vi "Attitude Control Test.vi"() -> ()   [LabVIEW 2022 SP3]
doc: "This example is used to make the attitude control"
uses:
  <vilib>/Utility/miscctls.llb/LV3DPointTypeDef.ctl
  lv-attitudecontrol.lvlib
panel:
  out "Numeric 3":dbl
  out "Numeric 2":dbl
  out "Numeric":dbl
  in  "Attitude Indicator":refnum<vi>(3d-picture)
  in  "stop":bool
  in  "Control 1":T1 {"X" scale=-90.0..90.0; "Y" scale=-180.0..180.0; "Z" scale=0.0..360.0}
  # "Overview: This example is used to make the attitude control\nRequirements: LabVIEW 2012 (or compatible)\nInstructions: \n1. Run this VI"
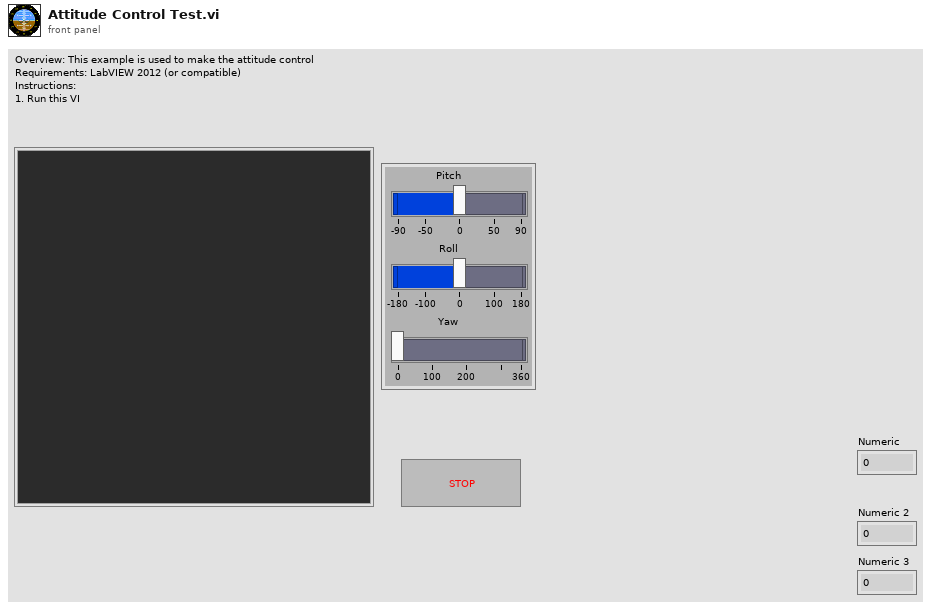
[diagram p1: front panel]
types:
  T1 = typedef "LV3DPointTypeDef.ctl" = cluster{"X":sgl, "Y":sgl, "Z":sgl}
  T2 = typedef "lv-attitudecontrol.lvlib/AttitudeHandle.ctl" = cluster{"First Scene Object":refnum<vi>, "Drum":refnum<vi>, "Window":refnum<vi>, "Dial":refnum<vi>, "Scene Graph":refnum<vi>, "Last Drum Pitch":dbl, "Last Drum Roll ":dbl, "Last Dial Roll":dbl}
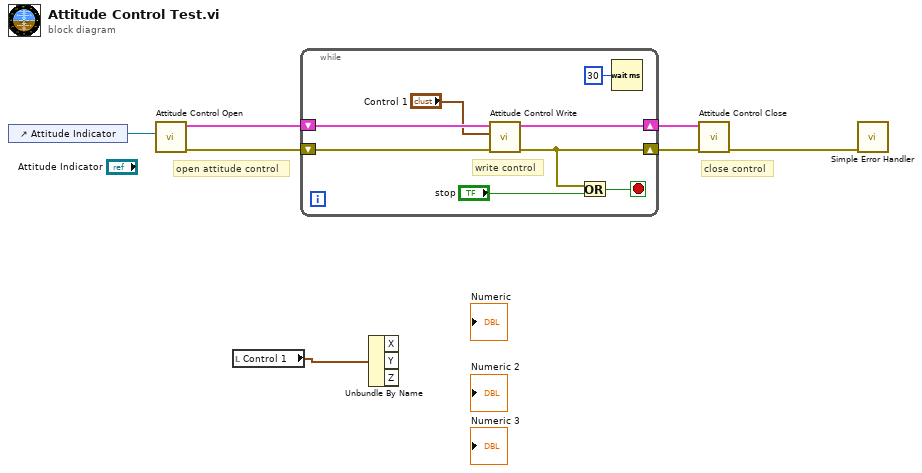
[diagram p0: block diagram]
diagram:
  # "close control"
  # "open attitude control"
  n1 = control-ref of="Attitude Indicator"() -> (w5:refnum<vi>)
  n2 = call "Attitude Control Open.vi"("Scene Graph"=w5) -> ("error out"=w6:errorcluster, "Attitude Control Handle"=w7:T2)  [unwired: 9 in]
  n3 = local read "Control 1"() -> (w1:T1)
  n4 = while {
    shift-right: [w8] -> w3
    shift-left: w7 -> [w15]
    shift-right: [w9] -> w4
    shift-left: w6 -> [w14]
    stop <- w10 stop-if-true
    # "write control"
    n5 = call "Attitude Control Write.vi"("error in (no error)"=w14, "pitch (x), roll (y), yaw (z)"="Control 1", "Attitude Control Handle In"=w15) -> ("error out"=w9:errorcluster, "Attitude Control Handle Out"=w8:T2)  [unwired: 7 in]
    n6 = Or(x=w9, y="stop") -> (x .or. y?=w10:bool)
    n7 = Wait (ms)(milliseconds to wait=u32 30) -> ()  [unwired: 1 out]
  }
  n8 = Unbundle By Name(w1) -> ()  [unwired: 3 out]
  n9 = call "Attitude Control Close.vi"("error in (no error)"=w4, "Attitude Control Handle"=w3) -> ("error out"=w2:errorcluster)  [unwired: 9 in]
  n10 = call <vilib>:"Simple Error Handler.vi"("error in (no error)"=w2) -> ()  [unwired: 4 in, 5 out]
